vi "RealSense_Test.vi"() -> ()   [LabVIEW 2023]
uses:
  support/Data-TypeDef.ctl
  support/Message Queue/Enqueue Message (Single).vi
  support/Message Queue/Message Queue.lvlib
  support/User Event - Stop/User Event - Stop.lvlib
panel:
  out "Output stream format":T1={"width"=1280, "height"=720, "fps"=30, "Profile"=605382696, "ppx"=634.5728, "ppy"=370.69974, "fx"=952.6064, "fy"=952.6064, "model"=4}
  in  "Color Presets":T2(ring)=enum."D435"
  in  "Depth Presets":T3(ring)=enum."Original"
  in  "laser on/off":bool=TRUE
  in  "autoexposure":bool=TRUE
  in  "Laser power, mW":sgl=150.0
  in  "Gain(16-248)":sgl=64.0
  in  "Exposure,us":sgl=156.0
  out "Depth map":sgl[][](graph)
  out "RGB image":picture
  out "iteration":i32=22
  in  "stop":bool=TRUE
  out "release frame error":string="No Error"
  out "Capture1 Error":string="No Error"
  out "Config error":string="No Error\rNo Error"
  out "init results":T4={"camera name"="Intel RealSense 415", "camera S/N"="725112060291", "F/W"="05.08.08.00", "Sensor name"="Stereo Module", "api_version"=20801, "rscontext"=606847696, "device_list"=597043920, "device count"=2, "Dev out"=606875504, "sensor_list"=605604656, "sensor count"=2, "Sensor out"=601640400}
  out "init error":string="No Error\rNo Error\rNo Error\rNo Error\rNo Error\rNo Error\rNo Error\rNo Error\rNo Error\rNo Error\rNo Error"
  out "Close Error":string="No Error\rNo Error\rNo Error\rNo Error"
  out "Start Error":string="No Error\rNo Error\rNo Error"
  out "Capture2 error":string="No Error"
  in  "Select Resolution":u16(ring)=15 items=["424 x 240 @6fps", "424 x 240 @15fps", "424 x 240 @30fps", "424 x 240 @60fps", "424 x 240 @90fps", "480 x 270 @6fps", "480 x 270 @15fps", "480 x 270 @30fps", "480 x 270 @60fps", "480 x 270 @90fps", "640 x 360 @6fps", "640 x 360 @15fps", "640 x 360 @30fps", "640 x 360 @60fps", "640 x 360 @90fps", "640 x 480 @6fps", "640 x 480 @15fps", "640 x 480 @30fps", "640 x 480 @60fps", "640 x 480 @90fps", "848 x 480 @6fps", "848 x 480 @15fps", "848 x 480 @30fps", "848 x 480 @60fps", "848 x 480 @90fps", "1280 x 720 @6fps", "1280 x 720 @15fps", "1280 x 720 @30fps"]
  # "RealSense Hello World: Color + Depth"
  # "This demo shows how to connect a RealSense D4xx Stereo Depth Camera, and stream the COLOR (left) and a DEPTH MAP."
  # "COLOR"
  # "DEPTH MAP"
  # "Note; When you change Depth Preset you need to stop and restart for the HDAD settings to take effect.\n\nTry the Color preset called \"Remove IR2\". It will remove the laser projector from the RGB 1280x720 image."
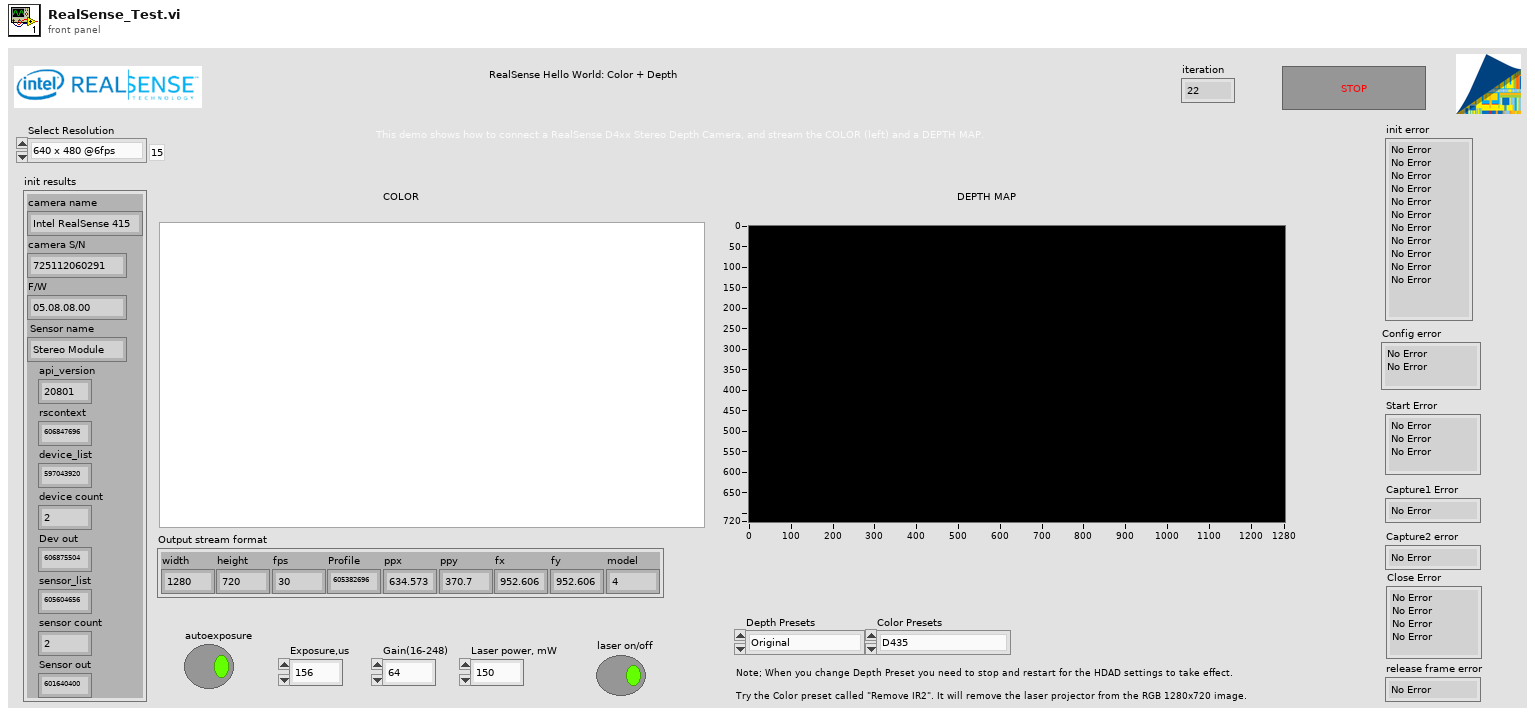
[diagram p1: front panel]
types:
  T1 = cluster{"width":i32, "height":i32, "fps":i32, "Profile":u64, "ppx":sgl, "ppy":sgl, "fx":sgl, "fy":sgl, "model":u32}
  T2 = enum16{"Custom", "RS400 (DS5p)", "RS400 (DS5p) 2", "RS400 (DS5p) 3", "RS400 (DS5p) 4", "RS400 (DS5p) 5", "RS410 (DS5a)", "RS410 (DS5a) 2", "DS410 (DS5a) 3", "DS410 (DS5a) 4", "DS410+IR", "DS5LR", "DS5LR-2", "DS5LR no pattern", "RS410 Remove IR", "RS410 Remove IR 2", "DS5micro", "D435"}
  T3 = enum16{"Custom", "Original", "New Depth 1", "New Depth 2", "Depth Active 1", "Active 3D Scan", "Active Short A", "Active Short C", "Face", "Face2", "Best Box", "High Density", "Medium Density", "High Accuracy", "Hand", "Short Range", "Flat wall", "Load .JSON", "Load .JSON2"}
  T4 = cluster{"camera name":string, "camera S/N":string, "F/W":string, "Sensor name":string, "api_version":i32, "rscontext":u64, "device_list":u64, "device count":i32, "Dev out":u64, "sensor_list":u64, "sensor count":i32, "Sensor out":u64}
  T5 = typedef "Data-TypeDef.ctl" = cluster{"Exposure (us)":sgl, "Gain (16-248)":sgl, "Laser Power (mW)":sgl, "Autoexposure":bool, "Laser":bool, "Color Presets":enum16{"Custom", "RS400 (DS5p)", "RS400 (DS5p) 2", "RS400 (DS5p) 3", "RS400 (DS5p) 4", "RS400 (DS5p) 5", "RS410 (DS5a)", "RS410 (DS5a) 2", "DS410 (DS5a) 3", "DS410 (DS5a) 4", "DS410+IR", "DS5LR", "DS5LR-2", "DS5LR no pattern", "RS410 Remove IR", "RS410 Remove IR 2", "DS5micro", "D435"}, "Depth Presets":enum16{"Custom", "Original", "New Depth 1", "New Depth 2", "Depth Active 1", "Active 3D Scan", "Active Short A", "Active Short C", "Face", "Face2", "Best Box", "High Density", "Medium Density", "High Accuracy", "Hand", "Short Range", "Flat wall", "Load .JSON", "Load .JSON2"}, "rscontext":u64, "dev":u64, "device_list":u64, "sensor":u64, "queue":u64}
  T6 = typedef "Message Queue.lvlib/All Message Queues.ctl" = cluster{"UI":refnum<queue>}
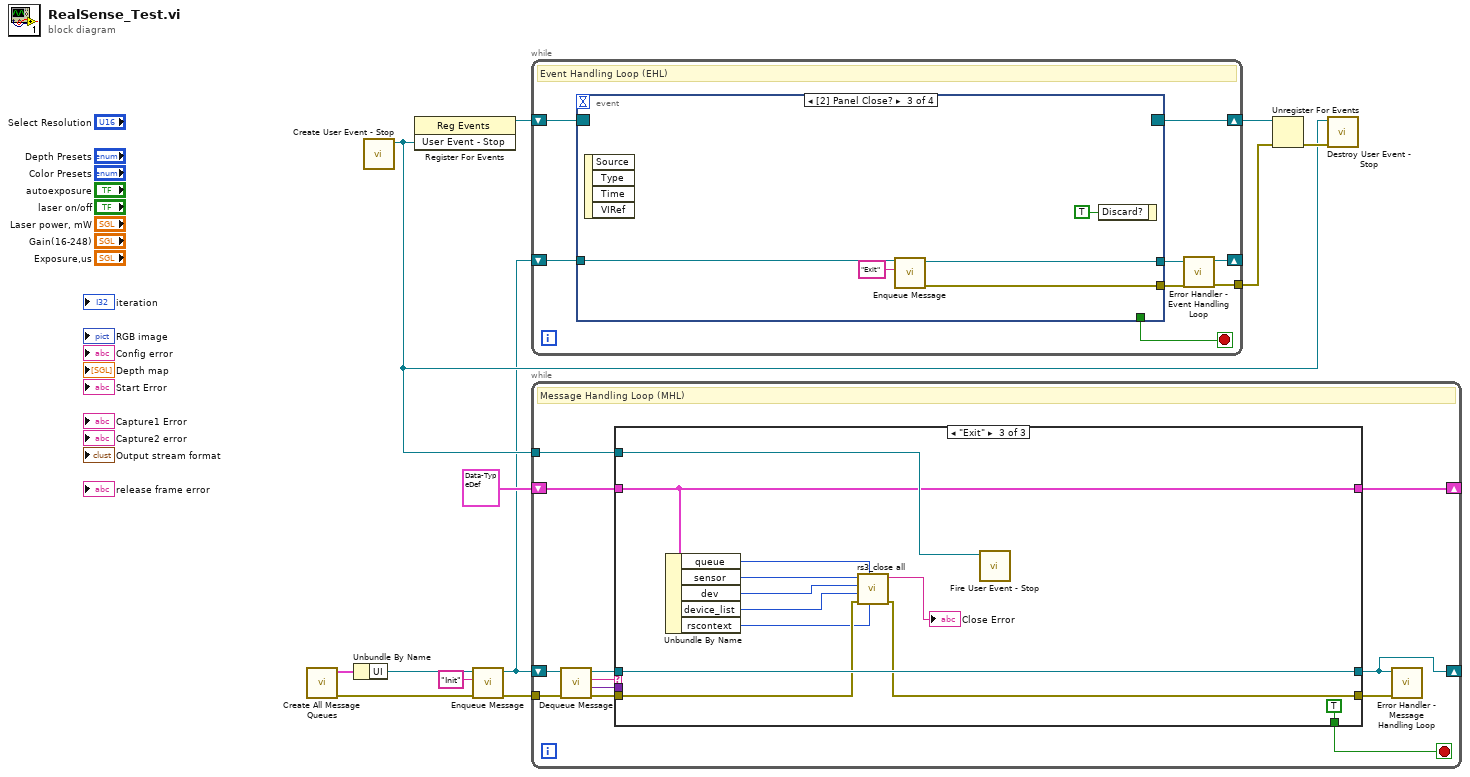
[diagram p0: block diagram]
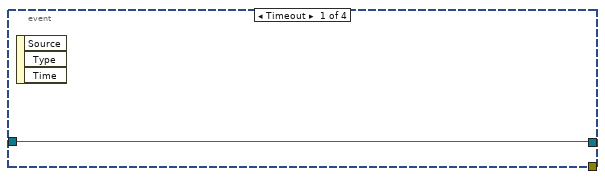
[diagram p2: hidden frame]
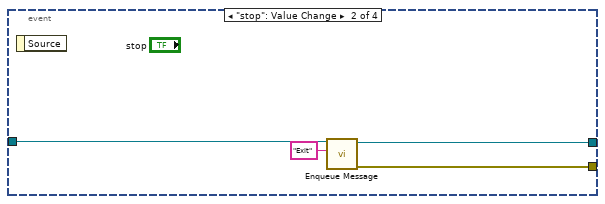
[diagram p3: hidden frame]
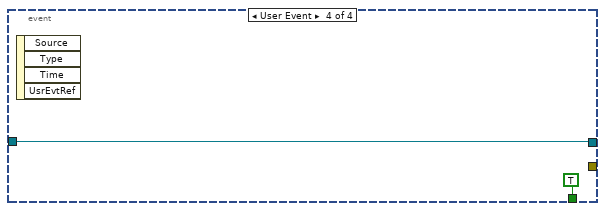
[diagram p4: hidden frame]
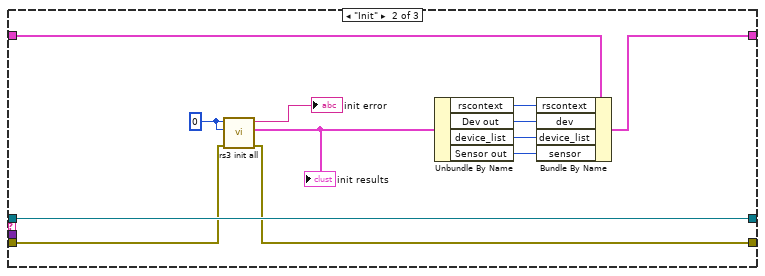
[diagram p6: hidden frame]
diagram:
  n1 = call "Create All Message Queues.vi"() -> ("error out"=w3:errorcluster, "Message Queues out"=w6:T6)  [unwired: 10 in]
  n2 = Unbundle By Name(w6) -> ("UI"=w5:refnum<queue>)
  n3 = call "Create User Event - Stop.vi"() -> ("User Event - Stop"=w8:refnum<user-event>)  [unwired: 10 in, 1 out]
  n4 = register-events(w8) -> (reference out=w12:refnum<event-registration>)  [unwired: 2 in, 1 out]
  n5 = call-poly "Enqueue Message.vi"("error in (no error)"=w3, "Message"="Init", "Message Queue"=w5) -> ("error out"=w2:errorcluster, "dup Message Queue"=w4:refnum<queue>)  [unwired: 7 in]
  n6 = while {
    shift-right: [w20] -> _
    shift-left: w4 -> [w19]
    shift-right: [w15] -> w10
    shift-left: w12 -> [w16]
    tunnel: [w13] -> w11
    stop <- w14 stop-if-true
    # "Event Handling Loop (EHL)"
    n7 = event shown="[2] Panel Close?" {
      selector: w16 -> [_ _ _ _]
      dyn-events: [_ _ _ _] -> w15
      timeout: _ -> [_ _ _ _]
      tunnel: w19 -> [w21 w25 w30 w31]
      tunnel: [w21 w23 w28 w31] -> w18
      tunnel: [_ w22 w27 _] -> w17
      tunnel: [_ _ _ TRUE] -> w14
      event Timeout {
        n8 = event-data() -> ()  [unwired: 1 in, 3 out]
      }
      event "stop": Value Change {
        n9 = event-data() -> ()  [unwired: 1 in, 1 out]
        n10 = call-poly "Enqueue Message.vi"("Message"="Exit", "Message Queue"=w25) -> ("error out"=w22:errorcluster, "dup Message Queue"=w23:refnum<queue>)  [unwired: 8 in]
      }
      event Panel Close? {
        n11 = event-data() -> ()  [unwired: 1 in, 4 out]
        n12 = call-poly "Enqueue Message.vi"("Message"="Exit", "Message Queue"=w30) -> ("error out"=w27:errorcluster, "dup Message Queue"=w28:refnum<queue>)  [unwired: 8 in]
        n13 = event-data("Discard?"=TRUE) -> ()  [unwired: 1 in, 1 out]
      }
      event User Event {
        n14 = event-data() -> ()  [unwired: 1 in, 4 out]
      }
    }
    n15 = call "Error Handler - Event Handling Loop.vi"("error in (no error)"=w17, "Message Queue"=w18) -> ("dup error in"=w13:errorcluster, "dup Message Queue"=w20:refnum<queue>)  [unwired: 8 in]
  }
  n16 = while {
    tunnel: w8 -> [w44]
    shift-right: [w40] -> _
    shift-left: w4 -> [w41]
    tunnel: w2 -> [w39]
    shift-right: [w33] -> _
    shift-left: T5 {"Exposure (us)"=0.0, "Gain (16-248)"=0.0, "Laser Power (mW)"=0.0, "Autoexposure"=FALSE, "Laser"=FALSE, "Color Presets"=enum."D435", "Depth Presets"=enum."Original", "rscontext"=606847696, "dev"=606875504, "device_list"=597043920, "sensor"=601640400, "queue"=601640400} ("Data") -> [w43]
    stop <- w34 stop-if-true
    # "Message Handling Loop (MHL)"
    n17 = call "Dequeue Message.vi"("error in (no error)"=w39, "Message Queue"=w41) -> ("error out"=w38:errorcluster, "Message Data"=w35:variant, "Message"=w36:string, "dup Message Queue"=w42:refnum<queue>)  [unwired: 6 in]
    n18 = case shown="\"Exit\"" w36 {
      tunnel: w44 -> [_ _ w69]
      tunnel: w43 -> [w47 w53 w68]
      tunnel: w42 -> [w46 w59 w71]
      tunnel: [w46 w59 w71] -> w40
      tunnel: w38 -> [w45 w58 w63]
      tunnel: [w45 w57 w62] -> w37
      tunnel: w35 -> [_ _ _]
      tunnel: [_ _ TRUE] -> w34
      tunnel: [w47 w48 w68] -> w33
      frame Default {
      }
      frame "Init" {
        w55 = 0 ("Select Sensor")
        n19 = call "rs3 init all.vi"("error in"=w58, "Select Device"=w55, "Select Sensor"=w55) -> ("error out"=w57:errorcluster, "init results"=w54:T4, "init error"=→"init error":string)  [unwired: 2 in, 4 out]
        "init results" <- w54
        n20 = Unbundle By Name(w54) -> ("rscontext"=w52:u64, "Dev out"=w51:u64, "device_list"=w50:u64, "Sensor out"=w49:u64)
        n21 = Bundle By Name(cluster=w53, "rscontext"=w52, "dev"=w51, "device_list"=w50, "sensor"=w49) -> (w48:T5)
      }
      frame "Exit" {
        n22 = Unbundle By Name(w68) -> ("queue"=w67:u64, "sensor"=w66:u64, "dev"=w65:u64, "device_list"=w64:u64, "rscontext"=w61:u64)
        n23 = call "rs3_close all.vi"("rscontext"=w61, "queue in"=w67, "error in (no error)"=w63, "device_list"=w64, "Dev in"=w65, "Sensor in"=w66) -> ("error out (no error)"=w62:errorcluster, "Close Error"=→"Close Error":string)  [unwired: 4 in]
        n24 = call "Fire User Event - Stop.vi"("User Event - Stop"=w69) -> ()  [unwired: 10 in, 1 out]
      }
    }
    n25 = call "Error Handler - Message Handling Loop.vi"("error in (no error)"=w37, "Message Queue"=w40) -> ()  [unwired: 8 in, 2 out]
  }
  n26 = Unregister For Events(event registration refnum=w10, error in=w11) -> (error out=w9:errorcluster)
  n27 = call "Destroy User Event - Stop.vi"("error in (no error)"=w9, "User Event - Stop"=w8) -> ()  [unwired: 9 in, 1 out]
